vi "TDMS Find Max Run Number.vi"(8 "error in (no error)":errorcluster, 11 "tdms file":refnum<k34>) -> (0 "error out":errorcluster, 1 "Max Run #":i32, 2 "Max Run Group ID":string, 3 "tdms file out":refnum<k34>, 5 "Next Run ID":string)   [LabVIEW 2011]
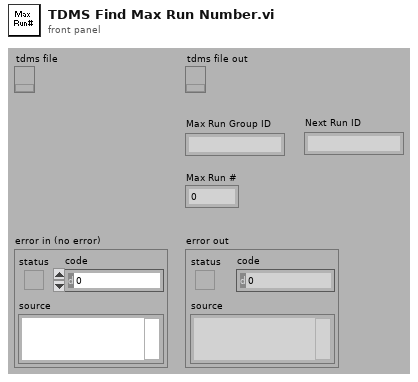
[diagram p1: front panel]
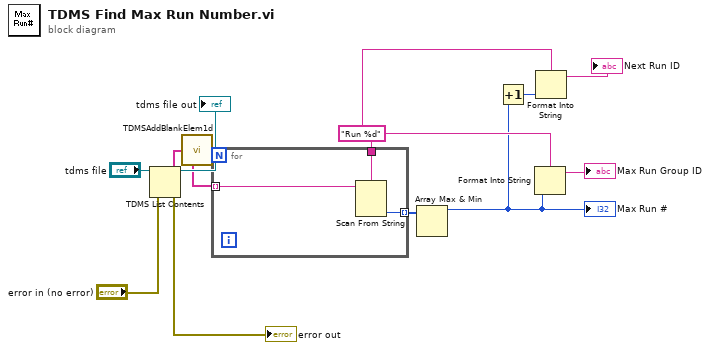
[diagram p0: block diagram]
diagram:
  w5 = "Run %d" ("format string")
  n1 = TDMS List Contents(4:"error in (no error)", 7:"tdms file") -> (0:→"error out":errorcluster, 2:w1:string[], 3:→"tdms file out":refnum<k34>)  [unwired: 2 out]
  n2 = call <vilib>:"TDMSAddBlankElem1d.vi"("input string array"=w1) -> ("output string array with blank element at the beginning"=w6:string[])
  n3 = for {
    tunnel: w6 -> [w14] mode=indexing
    tunnel: [w15] -> w12 mode=indexing
    tunnel: w5 -> [w13]
    n4 = Scan From String(format string=w13, input string=w14) -> (output 1=w15:i32)  [unwired: 2 in, 4 out]
  }
  n5 = Array Max & Min(array=w12) -> (max value=w2:i32)  [unwired: 3 out]
  "Max Run #" <- w2
  n6 = Increment(x=w2) -> (x+1=w4:i32)
  n7 = Format Into String(format string=w5, w2) -> (resulting string=→"Max Run Group ID":string)  [unwired: 2 in, 1 out]
  n8 = Format Into String(format string=w5, w4) -> (resulting string=→"Next Run ID":string)  [unwired: 2 in, 1 out]
